vi "CoverROI.vi"(8 "error in (no error)":errorcluster, 9 "Fitted Circle":T1, 10 "Matchs":T3(array[cluster]), 11 "Image":T2) -> (0 "error out":errorcluster, 3 "Image Out":T2)   [LabVIEW 2016]
uses:
  <vilib>/vision/Image Controls.llb/IMAQ Image.ctl
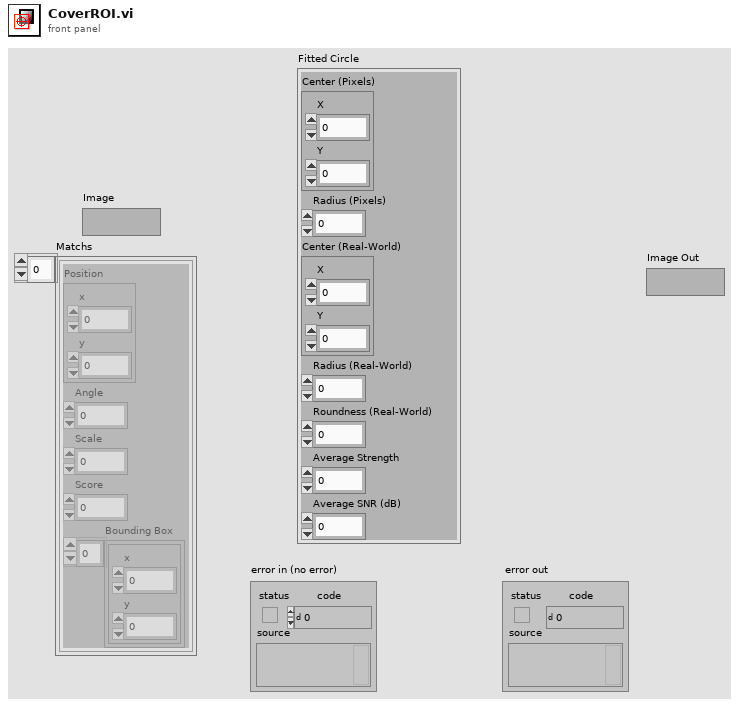
[diagram p1: front panel]
types:
  T1 = cluster{"Center (Pixels)":cluster{"X":sgl, "Y":sgl}, "Radius (Pixels)":dbl, "Center (Real-World)":cluster{"X":sgl, "Y":sgl}, "Radius (Real-World)":dbl, "Roundness (Real-World)":dbl, "Average Strength":dbl, "Average SNR (dB)":dbl}
  T2 = typedef "IMAQ Image.ctl" = refnum<image>
  T3 = cluster{"Position":cluster{"x":sgl, "y":sgl}, "Angle":sgl, "Scale":sgl, "Score":sgl, "Bounding Box":cluster{"x":sgl, "y":sgl}[]}[]
  T4 = typedef "IMAQ Circle" = cluster{"Center X":i32, "Center Y":i32, "Inner Radius":i32, "Outer Radius":i32, "Start Angle":dbl, "End Angle":dbl}
  T5 = cluster{"Position":cluster{"x":sgl, "y":sgl}, "Angle":sgl, "Scale":sgl, "Score":sgl, "Bounding Box":cluster{"x":sgl, "y":sgl}[]}
  T6 = typedef "ROI Descriptor" = cluster{"Global Rectangle":i32[], "Contours":cluster{"ID":enum32{"External", "Internal"}, "Type":u32, "Coordinates":i32[]}[]}
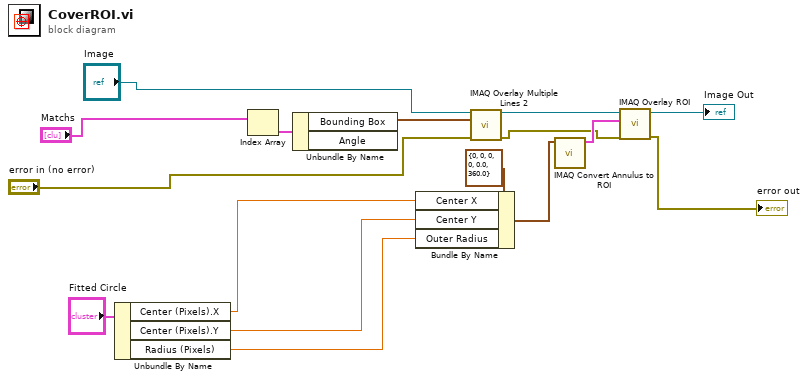
[diagram p0: block diagram]
diagram:
  n1 = Unbundle By Name("Fitted Circle") -> ("Center (Pixels).X"=w3:sgl, "Center (Pixels).Y"=w2:sgl, "Radius (Pixels)"=w1:dbl)
  n2 = Index Array(array="Matchs") -> (element=w16:T5)  [unwired: 1 in]
  n3 = Unbundle By Name(w16) -> ("Bounding Box"=w15:cluster{"x":sgl, "y":sgl}[])  [unwired: 1 out]
  n4 = Bundle By Name(cluster=T4 {"Center X"=0, "Center Y"=0, "Inner Radius"=0, "Outer Radius"=0, "Start Angle"=0.0, "End Angle"=360.0} ("Annulus"), "Center X"=w3, "Center Y"=w2, "Outer Radius"=w1) -> (w10:T4)
  n5 = call "IMAQ Overlay Multiple Lines 2"("Image"="Image", "Line End Points"=w15, "error in (no error)"="error in (no error)") -> ("Image Out"=w13:T2, "error out"=w7:errorcluster)  [unwired: 11 in]
  n6 = call "IMAQ Convert Annulus to ROI"("Annulus"=w10) -> ("ROI Descriptor"=w14:T6)  [unwired: 8 in, 1 out]
  n7 = call "IMAQ Overlay ROI"("error in (no error)"=w7, "ROI Descriptor"=w14, "Image"=w13) -> ("error out"=→"error out":errorcluster, "Image Out"=→"Image Out":T2)  [unwired: 7 in]
